vi "PID SP Limiter.vi"(7 "SpLim_State":T1, 8 "dt (s)":dbl=-1.0 format="%.2f", 9 "PV":dbl, 10 "SP":dbl, 11 "PID SP Limiter in":refnum<class "PID SP Limiter.lvclass">) -> (0 "dt (s) out":dbl, 1 "SpLim_State changed":bool, 2 "output":dbl format="%.2f", 3 "PID SP Limiter out":refnum<class "PID SP Limiter.lvclass">, 4 "pid_out_H":dbl format="%.2f")   [LabVIEW 2019, in "control.lvlib" / "PID SP Limiter.lvclass"]
uses:
  PID SP Limiter.lvclass
  D:/my_projects/projects/Algorithms/Labview/19/Reg/PID/PID Output Rate Limiter/PID Output Rate Limiter.lvclass
  ctl/SpLim_State.ctl
  PID SP Limiter.lvclass/PID SP Limiter.ctl
  PID Output Rate Limiter/PID Output Rate Limiter.lvclass/PID Output Rate Limiter.ctl
  PID Timing Estimation/PID Timing Estimation.lvclass/PID Timing Estimation.ctl
  PID Timing Estimation/PID Timing Estimation.vi
  PID Output Rate Limiter/PID Output Rate Limiter.lvclass
  D:/my_projects/projects/Algorithms/Labview/19/Reg/PID/PID Timing Estimation/PID Timing Estimation.lvclass
  control.lvlib
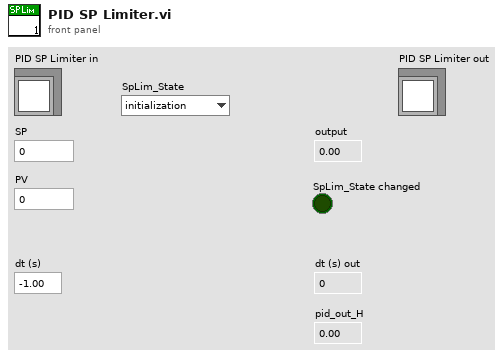
[diagram p1: front panel]
types:
  T1 = typedef "control.lvlib/SpLim_State.ctl" = enum8{"initialization", "stop", "decrease", "increase"}
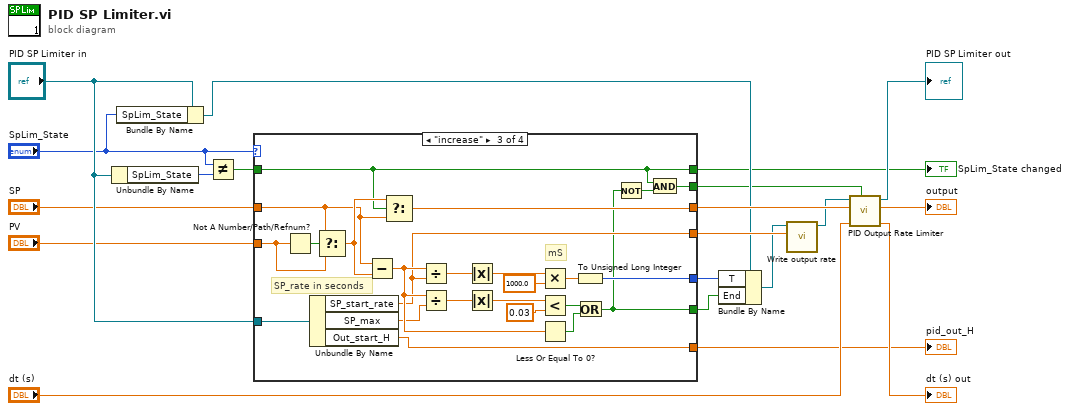
[diagram p0: block diagram]
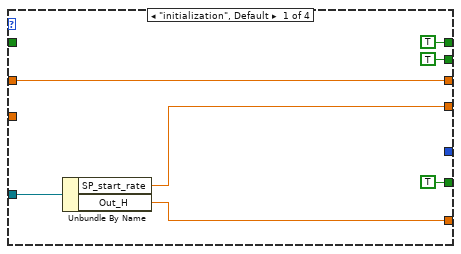
[diagram p2: hidden frame]
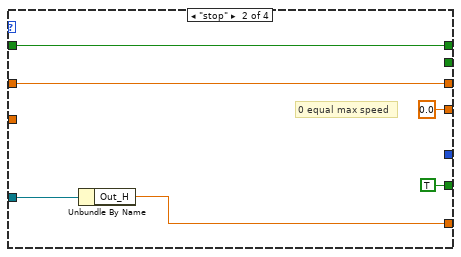
[diagram p3: hidden frame]
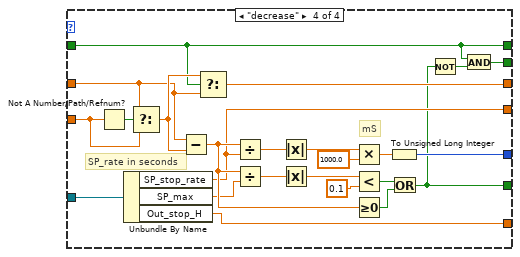
[diagram p4: hidden frame]
diagram:
  n1 = Unbundle By Name("PID SP Limiter in") -> ("SpLim_State"=w12:T1)
  n2 = Bundle By Name(cluster="PID SP Limiter in", "SpLim_State"="SpLim_State") -> (w7:refnum<class "PID SP Limiter.lvclass">)
  n3 = Not Equal?(x="SpLim_State", y=w12) -> (x != y?=w5:bool)
  n4 = case shown="\"increase\"" "SpLim_State" {
    tunnel: "SP" -> [w27 w33 w45 w69]
    tunnel: "PV" -> [_ _ w56 w80]
    tunnel: [w27 w33 w44 w71] -> w16
    tunnel: [_ _ w51 w74] -> w8
    tunnel: [TRUE TRUE w37 w62] -> w2
    tunnel: w5 -> [_ w29 w38 w63]
    tunnel: "PID SP Limiter in" -> [w26 w32 w52 w75]
    tunnel: [w23 0.0 ("SP_stop_rate") w42 w66] -> w13
    tunnel: [TRUE w29 w38 w63] -> w3
    tunnel: [w22 w30 w41 w65] -> w4
    tunnel: [TRUE _ w39 w61] -> w1
    frame "initialization", Default {
      n5 = Unbundle By Name(w26) -> ("SP_start_rate"=w23:dbl, "Out_H"=w22:dbl)
    }
    frame "stop" {
      # "0 equal max speed"
      n6 = Unbundle By Name(w32) -> ("Out_H"=w30:dbl)
    }
    frame "increase" {
      # "SP_rate in seconds"
      # "mS"
      n7 = Not A Number/Path/Refnum?(number/path/refnum=w56) -> (NaN/Path/Refnum?=w57:bool)
      n8 = Unbundle By Name(w52) -> ("SP_start_rate"=w42:dbl, "SP_max"=w43:dbl, "Out_start_H"=w41:dbl)
      n9 = Select(t=w45, s=w57, f=w56) -> (s? t:f=w46:dbl)
      n10 = Subtract(x=w45, y=w46) -> (x-y=w49:dbl)
      n11 = Select(t=w46, s=w38, f=w45) -> (s? t:f=w44:dbl)
      n12 = Divide(x=w49, y=w42) -> (x/y=w55:dbl)
      n13 = Divide(x=w49, y=w43) -> (x/y=w54:dbl)
      n14 = Absolute Value(x=w55) -> (abs(x)=w35:dbl)
      n15 = Absolute Value(x=w54) -> (abs(x)=w53:dbl)
      n16 = Multiply(x=w35, y=1000.0) -> (x*y=w36:dbl)
      n17 = Less?(x=w53, y=0.03) -> (x < y?=w48:bool)
      n18 = Less Or Equal To 0?(x=w49) -> (x <= 0?=w47:bool)
      n19 = To Unsigned Long Integer(number=w36) -> (unsigned 32bit integer=w51:u32)
      n20 = Or(x=w48, y=w47) -> (x .or. y?=w37:bool)
      n21 = Not(x=w37) -> (.not. x?=w40:bool)
      n22 = And(x=w38, y=w40) -> (x .and. y?=w39:bool)
    }
    frame "decrease" {
      # "SP_rate in seconds"
      # "mS"
      n23 = Not A Number/Path/Refnum?(number/path/refnum=w80) -> (NaN/Path/Refnum?=w81:bool)
      n24 = Unbundle By Name(w75) -> ("SP_stop_rate"=w66:dbl, "SP_max"=w67:dbl, "Out_stop_H"=w65:dbl)
      n25 = Select(t=w69, s=w81, f=w80) -> (s? t:f=w70:dbl)
      n26 = Subtract(x=w69, y=w70) -> (x-y=w68:dbl)
      n27 = Select(t=w70, s=w63, f=w69) -> (s? t:f=w71:dbl)
      n28 = Divide(x=w68, y=w66) -> (x/y=w79:dbl)
      n29 = Divide(x=w68, y=w67) -> (x/y=w78:dbl)
      n30 = Absolute Value(x=w79) -> (abs(x)=w58:dbl)
      n31 = Absolute Value(x=w78) -> (abs(x)=w77:dbl)
      n32 = Multiply(x=w58, y=1000.0) -> (x*y=w59:dbl)
      n33 = Less?(x=w77, y=0.1) -> (x < y?=w76:bool)
      n34 = Greater Or Equal To 0?(x=w68) -> (x >= 0?=w72:bool)
      n35 = To Unsigned Long Integer(number=w59) -> (unsigned 32bit integer=w74:u32)
      n36 = Or(x=w76, y=w72) -> (x .or. y?=w62:bool)
      n37 = Not(x=w62) -> (.not. x?=w64:bool)
      n38 = And(x=w63, y=w64) -> (x .and. y?=w61:bool)
    }
  }
  "SpLim_State changed" <- w3
  "pid_out_H" <- w4
  n39 = Bundle By Name(cluster=w7, "T"=w8, "End"=w2) -> (w6:refnum<class "PID SP Limiter.lvclass">)
  n40 = call "Write output rate.vi"("output rate"=w13, "PID Output Rate Limiter in"=w6) -> ("PID Output Rate Limiter out"=w14:refnum<class "PID SP Limiter.lvclass">)  [unwired: 9 in]
  n41 = call "PID Output Rate Limiter.vi"("reinitialize? (F)"=w1, "dt (s)"="dt (s)", "input (controller output)"=w16, "PID Output Rate Limiter in"=w14) -> ("dt (s) out"=→"dt (s) out":dbl, "output"=→"output":dbl, "PID Output Rate Limiter out"=→"PID SP Limiter out":refnum<class "PID SP Limiter.lvclass">)  [unwired: 5 in]
